vi "kvCanReadSync.vi"(2 "error in (no error)":errorcluster, 3 "Timeout":u32, 4 "Channel Handle (input only)":i32) -> (0 "error out":errorcluster, 1 "Channel Handle (ouput only)":i32)   [LabVIEW 2022 SP3]
doc: "Waits until the receive buffer contains at least one message or a timeout occurs."
uses:
  canlib32.dll
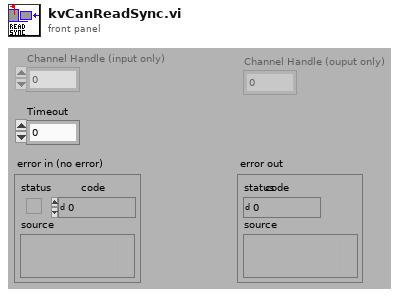
[diagram p1: front panel]
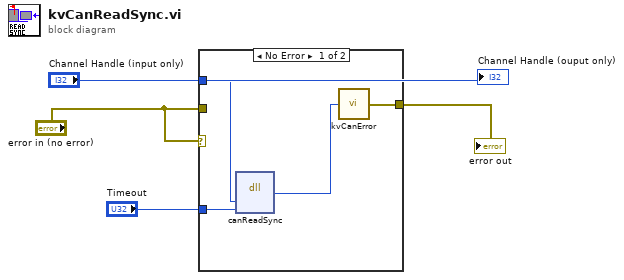
[diagram p0: block diagram]
diagram:
  n1 = case shown="No Error" "error in (no error)" {
    tunnel: "error in (no error)" -> [_ w9]
    tunnel: "Channel Handle (input only)" -> [w7 _]
    tunnel: [w6 w9] -> w2
    tunnel: "Timeout" -> [w5 _]
    frame No Error {
      n2 = dll-call lib="canlib32.dll" fn="canReadSync" label="Call CanReadSync"("channelHandle"=w7, "timeout"=w5) -> (w8:i32)  [unwired: 5 in, 2 out]
      n3 = call "kvCanError.vi"("error code"=w8) -> ("error out"=w6:errorcluster)
    }
    frame Error {
    }
  }
  "error out" <- w2
  "Channel Handle (ouput only)" <- "Channel Handle (input only)"
